vi "filter tags by writer.vi"(10 "exceptions":string[](array[string]), 11 "engine configuration in":refnum<class "engine configuration.lvclass">) -> (2 "tag list":refnum<class "tag descriptor.lvclass">[](array[class]), 3 "engine configuration out":refnum<class "engine configuration.lvclass">)   [LabVIEW 2013, in "engine configuration.lvclass"]
uses:
  engine configuration.lvclass
  <vilib>/NI/Tag Bus/tag/tag descriptor.lvclass
  engine configuration.lvclass/engine configuration.ctl
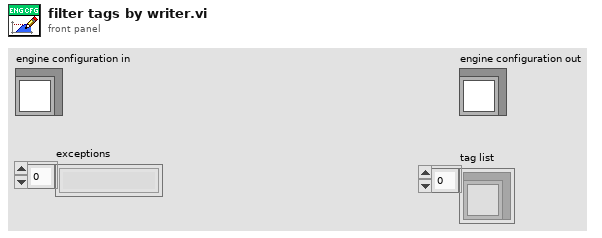
[diagram p1: front panel]
types:
  T1 = typedef "engine configuration.lvclass/Tag Info.ctl" = cluster{"Tag":refnum<class "tag descriptor.lvclass">, "Writer":string, "Readers":string[], "Owning ID":string}
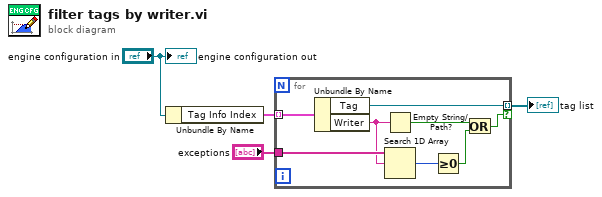
[diagram p0: block diagram]
diagram:
  n1 = Unbundle By Name("engine configuration in") -> ("Tag Info Index"=w3:T1[])
  n2 = for {
    tunnel: w3 -> [w12] mode=indexing
    tunnel: [w11] -> w2 mode=indexing if=w6
    tunnel: "exceptions" -> [w9]
    n3 = Unbundle By Name(w12) -> ("Tag"=w11:refnum<class "tag descriptor.lvclass">, "Writer"=w8:string)
    n4 = Empty String/Path?(string/path=w8) -> (empty?=w10:bool)
    n5 = Search 1D Array(1D array=w9, element=w8) -> (index of element=w7:i32)  [unwired: 1 in]
    n6 = Greater Or Equal To 0?(x=w7) -> (x >= 0?=w5:bool)
    n7 = Or(x=w10, y=w5) -> (x .or. y?=w6:bool)
  }
  "tag list" <- w2
  "engine configuration out" <- "engine configuration in"
